vi "steval-mki172V1_testing.vi"   [LabVIEW 2019]
uses:
  <vilib>/eio/EIONode/EIONode.xnode
  <vilib>/rvi/eio/common/nirviEmuTemplateMethod_errors.vi
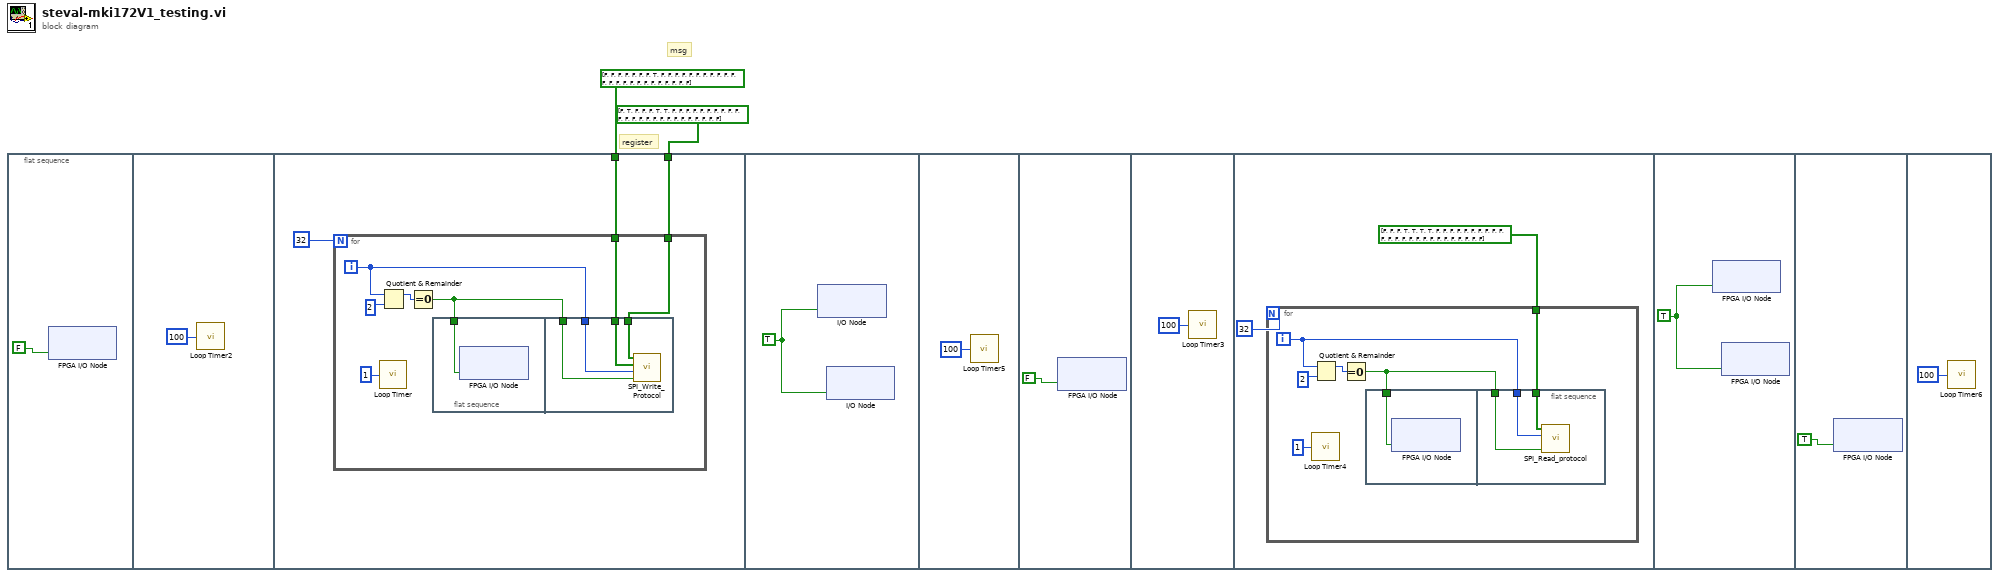
[diagram p0: block diagram]
diagram:
  # "register"
  # "msg"
  n1 = flat-sequence {
    tunnel: bool[] [FALSE, FALSE, FALSE, FALSE, FALSE, FALSE, FALSE, TRUE, FALSE, FALSE, FALSE, FALSE, FALSE, FALSE, FALSE, FALSE, FALSE, FALSE, FALSE, FALSE, FALSE, FALSE, FALSE, FALSE, FALSE, FALSE, FALSE, FALSE, FALSE, FALSE, FALSE, FALSE] ("message") -> [w6]
    tunnel: bool[] [FALSE, TRUE, FALSE, FALSE, FALSE, TRUE, TRUE, FALSE, FALSE, FALSE, FALSE, FALSE, FALSE, FALSE, FALSE, FALSE, FALSE, FALSE, FALSE, FALSE, FALSE, FALSE, FALSE, FALSE, FALSE, FALSE, FALSE, FALSE, FALSE, FALSE, FALSE, FALSE] ("Register_adress") -> [w5]
    frame #0 {
      n2 = xnode "FPGA I/O Node"("CS"=FALSE) -> ()  [unwired: 1 in, 1 out]
    }
    frame #1 {
      n3 = call "Loop Timer2"("Count(uSec)"=u32 100 ("Count(Ticks)")) -> ()  [unwired: 1 out]
    }
    frame #2 {
      n4 = for {
        N: 32 -> [_]
        tunnel: w6 -> [w9]
        tunnel: w5 -> [w8]
        i -> [w10]
        n5 = call "Loop Timer"("Count(mSec)"=u32 1) -> ()  [unwired: 1 out]
        n6 = Quotient & Remainder(x=w10, y=2) -> (x-y*floor(x/y)=w13:i32)  [unwired: 1 out]
        n7 = Equal To 0?(x=w13) -> (x = 0?=w11:bool)
        n8 = flat-sequence {
          tunnel: w11 -> [w15]
          tunnel: w11 -> [w16]
          tunnel: w10 -> [w17]
          tunnel: w9 -> [w19]
          tunnel: w8 -> [w18]
          frame #0 {
            n9 = xnode "FPGA I/O Node"("SCL"=w15) -> ()  [unwired: 1 in, 1 out]
          }
          frame #1 {
            n10 = call "SPI_Write_Protocol.vi"("rising_edge"=w16, "bit_index"=w17, "message"=w19, "Register_adress"=w18) -> ()  [unwired: 8 in]
          }
        }
      }
    }
    frame #3 {
      w20 = TRUE ("CS")
      n11 = xnode "I/O Node"("CS"=w20) -> ()  [unwired: 1 in, 1 out]
      n12 = xnode "I/O Node"("SCL"=w20) -> ()  [unwired: 1 in, 1 out]
    }
    frame #4 {
      n13 = call "Loop Timer5"("Count(uSec)"=u32 100 ("Count(Ticks)")) -> ()  [unwired: 1 out]
    }
    frame #5 {
      n14 = xnode "FPGA I/O Node"("CS"=FALSE) -> ()  [unwired: 1 in, 1 out]
    }
    frame #6 {
      n15 = call "Loop Timer3"("Count(uSec)"=u32 100 ("Count(Ticks)")) -> ()  [unwired: 1 out]
    }
    frame #7 {
      n16 = for {
        N: 32 -> [_]
        tunnel: bool[] [FALSE, FALSE, FALSE, TRUE, TRUE, TRUE, TRUE, FALSE, FALSE, FALSE, FALSE, FALSE, FALSE, FALSE, FALSE, FALSE, FALSE, FALSE, FALSE, FALSE, FALSE, FALSE, FALSE, FALSE, FALSE, FALSE, FALSE, FALSE, FALSE, FALSE, FALSE, FALSE] ("Register_adress") -> [w26]
        i -> [w27]
        n17 = call "Loop Timer4"("Count(mSec)"=u32 1) -> ()  [unwired: 1 out]
        n18 = Quotient & Remainder(x=w27, y=2) -> (x-y*floor(x/y)=w30:i32)  [unwired: 1 out]
        n19 = Equal To 0?(x=w30) -> (x = 0?=w28:bool)
        n20 = flat-sequence {
          tunnel: w28 -> [w32]
          tunnel: w28 -> [w35]
          tunnel: w27 -> [w34]
          tunnel: w26 -> [w33]
          frame #0 {
            n21 = xnode "FPGA I/O Node"("SCL"=w32) -> ()  [unwired: 1 in, 1 out]
          }
          frame #1 {
            n22 = call "SPI_Read_protocol.vi"("Register_adress"=w33, "bit_index"=w34, "rising_edge"=w35) -> ()  [unwired: 6 in, 1 out]
          }
        }
      }
    }
    frame #8 {
      w36 = TRUE ("CS")
      n23 = xnode "FPGA I/O Node"("CS"=w36) -> ()  [unwired: 1 in, 1 out]
      n24 = xnode "FPGA I/O Node"("SCL"=w36) -> ()  [unwired: 1 in, 1 out]
    }
    frame #9 {
      n25 = xnode "FPGA I/O Node"("CS"=TRUE) -> ()  [unwired: 1 in, 1 out]
    }
    frame #10 {
      n26 = call "Loop Timer6"("Count(uSec)"=u32 100 ("Count(Ticks)")) -> ()  [unwired: 1 out]
    }
  }
